vi "main.vi"() -> ()   [LabVIEW 2016]
panel:
  in  "Sampling Rate (Hz)":u32=10
  out "Threshold":dbl
  out "Muscle Signal":cluster{"Y":dbl[], "Y":dbl[]}[](graph)
  out "Max Muscle Power":sgl
  out "Max Duration":dbl
  in  "stop":bool
  out "Total Contraction TImes":dbl
  in  "Virtual Key":u8(ring)=32
  out "Current Duration":dbl
  out "Total Duration":dbl
  out "Current Muscle Power":sgl
  # "Instructions:\n1. Type in the Sampling Rate (recommend 10~30Hz).\n2. Choose the key or mouse action you want to simulate.\n3. Run the program.\n4. Calibrate your muscle sensor in the pop-up window.\n5. Open the game you want to play and enjoy! ^-^"
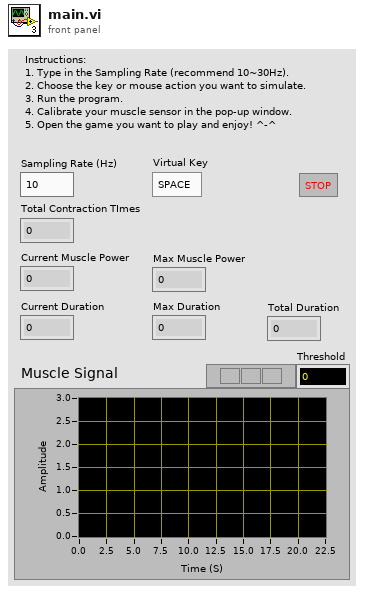
[diagram p1: front panel]
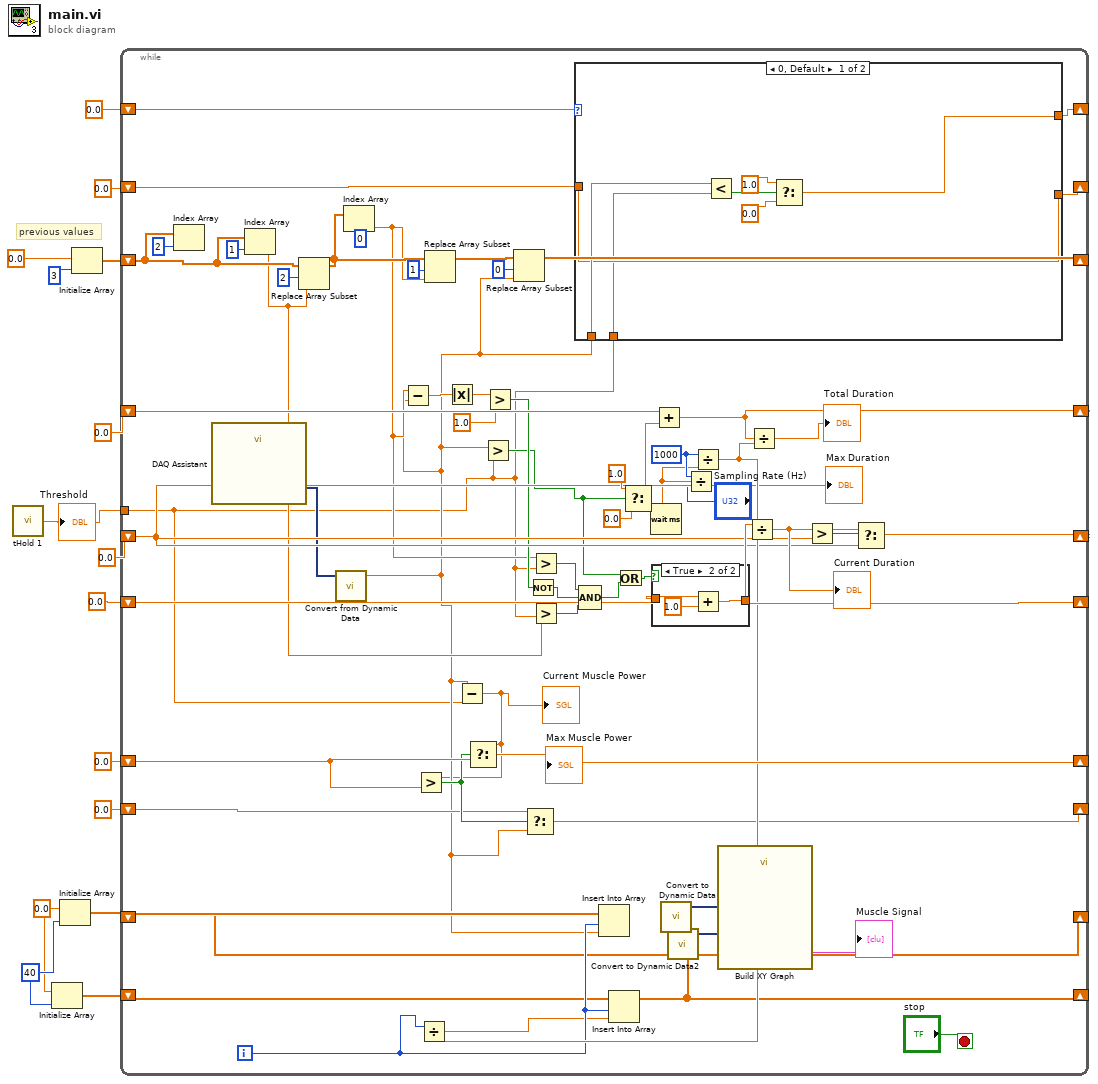
[diagram p0: block diagram]
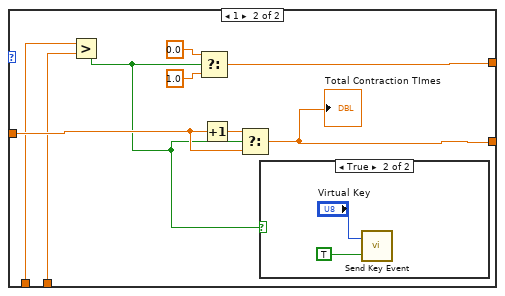
[diagram p2: hidden frame]
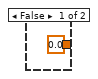
[diagram p4: hidden frame]
diagram:
  w9 = 40 ("dimension size")
  w8 = 0.0 ("element")
  # "previous values"
  n1 = call "tHold 1.vi"() -> ("My Threshold"=w3:dbl)  [unwired: 2 in]
  "Threshold" <- w3
  n2 = Initialize Array(w8, w9) -> (w7:dbl[])
  n3 = Initialize Array(w8, w9) -> (w10:dbl[])
  n4 = Initialize Array(0.0 ("element"), 3 ("dimension size")) -> (w4:dbl[])
  n5 = while {
    shift-right: [w71] -> _
    shift-left: 0.0 -> [w45]
    shift-right: [w70] -> _
    shift-left: 0.0 -> [w69]
    shift-right: [w66] -> _
    shift-left: 0.0 ("f") -> [w67]
    shift-right: [w65] -> _
    shift-left: 0.0 -> [w68]
    shift-right: [w63] -> _
    shift-left: 0.0 -> [w46]
    shift-right: [w61] -> _
    shift-left: 0.0 -> [w62]
    shift-right: [w53] -> _
    shift-left: w10 -> [w60]
    shift-right: [w55] -> _
    shift-left: w7 -> [w57]
    shift-right: [w49] -> _
    shift-left: 0.0 ("Scalar") -> [w47]
    shift-right: [w28] -> _
    shift-left: w4 -> [w26]
    tunnel: w3 -> [w20]
    i -> [w58]
    stop <- "stop" stop-if-true
    w18 = u32 1000 ("x")
    n6 = Index Array(array=w26, index=2) -> ()  [unwired: 1 out]
    n7 = call "DAQ Assistant"() -> ("data"=w22:dynamicdata)  [unwired: 17 in, 2 out]
    n8 = Index Array(array=w26, index=1) -> (element=w25:dbl)
    n9 = Replace Array Subset(array=w26, new element=w25, index=2) -> (w29:dbl[])
    n10 = call "Convert from Dynamic Data"("Dynamic Data Type"=w22) -> ("Scalar"=w21:dbl)  [unwired: 3 in]
    n11 = Index Array(array=w29, index=0) -> (element=w23:dbl)
    n12 = Subtract(x=w23, y=w21) -> (x-y=w44:dbl)
    n13 = Replace Array Subset(array=w29, new element=w23, index=1) -> (w32:dbl[])
    n14 = Absolute Value(x=w44) -> (abs(x)=w43:dbl)
    n15 = Subtract(x=w21, y=w20) -> (x-y=w19:dbl)
    "Current Muscle Power" <- w19
    n16 = Greater?(x=w19, y=w62) -> (0:w48:bool)
    n17 = Select(t=w19, s=w48, f=w62) -> (s? t:f=w61:dbl)
    "Max Muscle Power" <- w61
    n18 = Greater?(x=w21, y=w20) -> (0:w38:bool)
    n19 = Greater?(x=w43, y=1.0) -> (0:w41:bool)
    n20 = Replace Array Subset(array=w32, new element=w21, index=0) -> (w28:dbl[])
    n21 = Select(t=w47, s=w48, f=w21) -> (s? t:f=w49:dbl)
    n22 = Not(x=w41) -> (.not. x?=w36:bool)
    n23 = Greater?(x=w23, y=w20) -> (0:w40:bool)
    n24 = Greater?(x=w25, y=w20) -> (0:w24:bool)
    n25 = case shown="0, Default" w67 {
      tunnel: w68 -> [w79 w89]
      tunnel: w21 -> [w80 w88]
      tunnel: [w79 w87] -> w65
      tunnel: [w78 w86] -> w66
      tunnel: w20 -> [w77 w85]
      frame 0, Default {
        n26 = Less?(x=w80, y=w77) -> (x < y?=w81:bool)
        n27 = Select(t=1.0, s=w81, f=0.0) -> (s? t:f=w78:dbl)
      }
      frame 1 {
        n28 = Greater?(x=w88, y=w85) -> (0:w84:bool)
        n29 = Select(t=0.0, s=w84, f=1.0) -> (s? t:f=w86:dbl)
        n30 = Increment(x=w89) -> (x+1=w90:dbl)
        n31 = Select(t=w90, s=w84, f=w89) -> (s? t:f=w87:dbl)
        "Total Contraction TImes" <- w87
        n32 = case shown="True" w84 {
          frame False {
          }
          frame True {
            n33 = call "Send Key Event.vi"("(t)Press (f)Release"=TRUE, "Virtual Key"="Virtual Key") -> ()  [unwired: 1 out]
          }
        }
      }
    }
    n34 = Compound Arithmetic op=AND(w40, w36, w24) -> (w39:bool)
    n35 = Insert Into Array(array=w60, index=w58, new element=w21) -> (w53:dbl[])
    n36 = Or(x=w38, y=w39) -> (x .or. y?=w37:bool)
    n37 = Select(t=1.0, s=w38, f=0.0) -> (s? t:f=w73:dbl)
    n38 = case shown="True" w37 {
      tunnel: [0.0 w97] -> w70
      tunnel: w69 -> [_ w96]
      frame False {
      }
      frame True {
        n39 = Add(x=w96, y=1.0) -> (x+y=w97:dbl)
      }
    }
    n40 = Add(x=w45, y=w73) -> (x+y=w71:dbl)
    n41 = call "Convert to Dynamic Data2"("Array"=w53) -> ("Dynamic Data Type"=w52:dynamicdata)  [unwired: 3 in]
    n42 = Divide(x=w18, y="Sampling Rate (Hz)") -> (x/y=w16:dbl)
    n43 = Wait (ms)(milliseconds to wait=w16) -> ()  [unwired: 1 out]
    n44 = Divide(x=w18, y=w16) -> (x/y=w59:dbl)
    n45 = Divide(x=w58, y=w59) -> (x/y=w56:dbl)
    n46 = Insert Into Array(array=w57, index=w58, new element=w56) -> (w55:dbl[])
    n47 = call "Convert to Dynamic Data"("Array"=w55) -> ("Dynamic Data Type"=w54:dynamicdata)  [unwired: 3 in]
    n48 = call "Build XY Graph"("Y Input"=w52, "X Input"=w54) -> ("XY Graph"=→"Muscle Signal":cluster{"X":dbl[], "Y":dbl[]}[])  [unwired: 8 in, 1 out]
    n49 = Divide(x=w70, y=w59) -> (x/y=w64:dbl)
    "Current Duration" <- w64
    n50 = Divide(x=w71, y=w59) -> (x/y=→"Total Duration":dbl)
    n51 = Greater?(x=w64, y=w46) -> (0:w50:bool)
    n52 = Select(t=w64, s=w50, f=w46) -> (s? t:f=w63:dbl)
    "Max Duration" <- w46
  }
